vi "MotorValue.vi"() -> ()   [LabVIEW 2015]
panel:
  in  "Boolean":bool
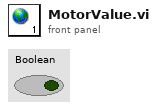
[diagram p1: front panel]
diagram:
